vi "Main.vi"() -> ()   [LabVIEW 2020]
uses:
  SubModules/AddModule.lvlibp
  SubModules/DivideModule.lvlibp
  SubModules/SubtractModule.lvlibp
  SubModules/MultipleModule.lvlibp
panel:
  out "Result":dbl
  in  "Function":enum16{"Add", "Subtract", "Multiple", "Divide"}(ring)
  in  "Y":dbl=2.0
  in  "X":dbl=4.0
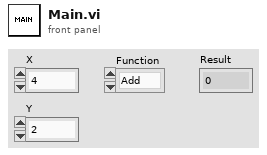
[diagram p1: front panel]
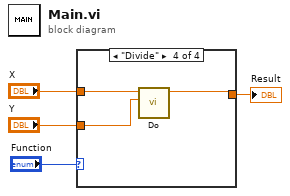
[diagram p0: block diagram]
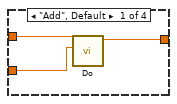
[diagram p2: hidden frame]
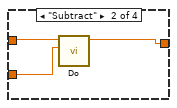
[diagram p3: hidden frame]
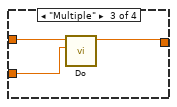
[diagram p4: hidden frame]
diagram:
  n1 = case shown="\"Divide\"" "Function" {
    tunnel: "X" -> [w7 w10 w13 w16]
    tunnel: "Y" -> [w6 w9 w12 w15]
    tunnel: [w5 w8 w11 w14] -> w1
    frame "Add", Default {
      n2 = call "Do.vi"("Y"=w6, "X"=w7) -> ("Result"=w5:dbl)  [unwired: 9 in]
    }
    frame "Subtract" {
      n3 = call "Do.vi"("Y"=w9, "X"=w10) -> ("Result"=w8:dbl)  [unwired: 9 in]
    }
    frame "Multiple" {
      n4 = call "Do.vi"("Y"=w12, "X"=w13) -> ("Result"=w11:dbl)  [unwired: 9 in]
    }
    frame "Divide" {
      n5 = call "Do.vi"("Y"=w15, "X"=w16) -> ("Result"=w14:dbl)  [unwired: 9 in]
    }
  }
  "Result" <- w1
